vi "_AttachCHK.vi"(8 "error in":errorcluster, 11 "Device In":i32) -> (0 "error out":errorcluster, 2 "Attached?":bool, 3 "Device Out":i32)   [LabVIEW 2014]
uses:
  phidget21.dll
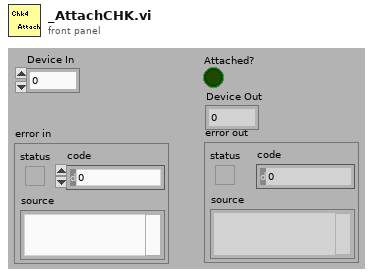
[diagram p1: front panel]
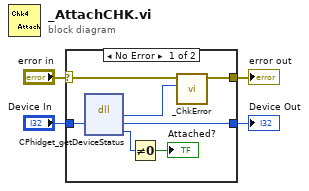
[diagram p0: block diagram]
diagram:
  n1 = case shown="No Error" "error in" {
    selector: "error in" -> [w7 w13]
    tunnel: [w6 w13] -> w3
    tunnel: [w10 w12] -> w2
    tunnel: "Device In" -> [w11 w12]
    frame No Error {
      n2 = dll-call lib="phidget21.*" fn="CPhidget_getDeviceStatus"("phid"=w11) -> (w5:i32, "phid"=w10:i32, "deviceStatus"=w9:i32)  [unwired: 4 in, 2 out]
      n3 = Not Equal To 0?(x=w9) -> (x != 0?=→"Attached?":bool)
      n4 = call "_ChkError.vi"("Return Code"=w5, "error in (no error)"=w7) -> ("error out"=w6:errorcluster)  [unwired: 9 in]
    }
    frame Error {
    }
  }
  "error out" <- w3
  "Device Out" <- w2
